vi "END.vi"(1 "Numeric":dbl) -> (0 "number":u32)   [LabVIEW 2014]
panel:
  in  "?":cluster{"OK Button":bool, "OK Button 2":bool}
  out "String":string
  # "得分:"
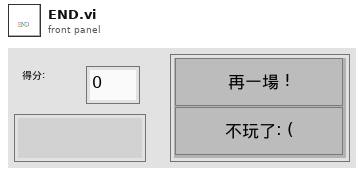
[diagram p1: front panel]
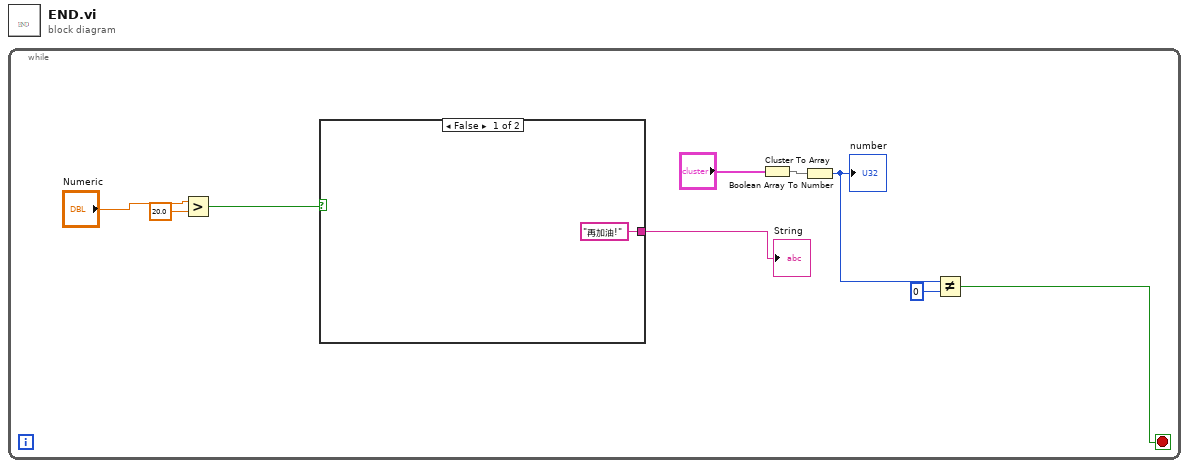
[diagram p0: block diagram]
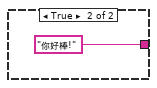
[diagram p2: hidden frame]
diagram:
  n1 = while {
    stop <- w1 stop-if-true
    n2 = Greater?(x="Numeric", y=20.0) -> (0:w7:bool)
    n3 = case shown="False" w7 {
      tunnel: ["再加油!" ("String") "你好棒!" ("String")] -> w6
      frame False {
      }
      frame True {
      }
    }
    "String" <- w6
    n4 = Cluster To Array(cluster="?") -> (array=w4:bool[])
    n5 = Boolean Array To Number(Boolean array=w4) -> (number=w3:u32)
    "number" <- w3
    n6 = Not Equal?(x=w3, y=u32 0) -> (x != y?=w1:bool)
  }
